vi "AIT 1553 - ReadWrite All Data.vi"(5 "Bus Section":T1, 6 "Iteration":i32, 7 "Mode":T2, 8 "error in (no error)":errorcluster, 11 "RT Data in":T3 {"Acyclic Frame Refs" format="%.0x"; "Label Transfer Config"."Block Data Refs"."Data Reference" format="%.0x"; "Status Config"."HWOut Dur Ref" format="%.0x"; "Status Config"."HWIn Dur Ref" format="%.0x"; "Status Config"."HWOut Count Ref" format="%.0x"; "Status Config"."HWIn Count Ref" format="%.0x"; "Status Config"."Error Data Ref" format="%.0x"; "HWOutput Channels"."Message Settings"."Driver Data"."First Word" min=8 max=31; "HWOutput Channels"."Message Settings"."Driver Data"."Num Bits" min=1 max=32; "HWOutput Channels"."Message Settings"."Driver Data"."Start Bit" min=8 max=31; "HWOutput Channels"."Message Settings"."Block Data Refs"."Data Reference" format="%.0x"; "HWInput Channels"."Message Settings"."Driver Data"."First Word" min=8 max=31; "HWInput Channels"."Message Settings"."Driver Data"."Num Bits" min=1 max=32; "HWInput Channels"."Message Settings"."Driver Data"."Start Bit" min=8 max=31; "HWInput Channels"."Message Settings"."Block Data Refs"."Data Reference" format="%.0x"}) -> (0 "error out":errorcluster, 3 "RT Data out":T3 {"Acyclic Frame Refs" format="%.0x"; "Label Transfer Config"."Block Data Refs"."Data Reference" format="%.0x"; "Status Config"."HWOut Dur Ref" format="%.0x"; "Status Config"."HWIn Dur Ref" format="%.0x"; "Status Config"."HWOut Count Ref" format="%.0x"; "Status Config"."HWIn Count Ref" format="%.0x"; "Status Config"."Error Data Ref" format="%.0x"; "HWOutput Channels"."Message Settings"."Driver Data"."First Word" min=8 max=31; "HWOutput Channels"."Message Settings"."Driver Data"."Num Bits" min=1 max=32; "HWOutput Channels"."Message Settings"."Driver Data"."Start Bit" min=8 max=31; "HWOutput Channels"."Message Settings"."Block Data Refs"."Data Reference" format="%.0x"; "HWInput Channels"."Message Settings"."Driver Data"."First Word" min=8 max=31; "HWInput Channels"."Message Settings"."Driver Data"."Num Bits" min=1 max=32; "HWInput Channels"."Message Settings"."Driver Data"."Start Bit" min=8 max=31; "HWInput Channels"."Message Settings"."Block Data Refs"."Data Reference" format="%.0x"})   [LabVIEW 2013, in "AIT 1553 Custom Device.lvlib"]
uses:
  AIT 1553 Custom Device.lvlib
  RT Controls/AIT 1553  - RT Data.ctl
  RT Controls/AIT 1553 - RT HW Channel.ctl
  RT Controls/AIT 1553 - Bus Section.ctl
  RT Controls/AIT 1553 - RT Message Settings.ctl
  <vilib>/NI Veristand/Custom Device API/Block Data Reference.ctl
  <vilib>/NI Veristand/Custom Device API/Data Reference.ctl
  RT Controls/AIT 1553 - Driver Data.ctl
  Controls and Global/Start Bit.ctl
  Controls and Global/Number of Bits.ctl
  RT Controls/AIT 1553 - Board Config Info.ctl
  RT Controls/AIT 1553 - Hardware Type.ctl
  RT Controls/Error Qs.ctl
  RT Controls/Status Channels Config.ctl
  RT Controls/FIFO.ctl
  RT Controls/Label Transfer Config.ctl
  <vilib>/NI Veristand/Custom Device API/Custom Device Item Ref.ctl
  RT Controls/ReadWrite Selector.ctl
  <vilib>/NI Veristand/Custom Device API/Custom Device API.lvlib
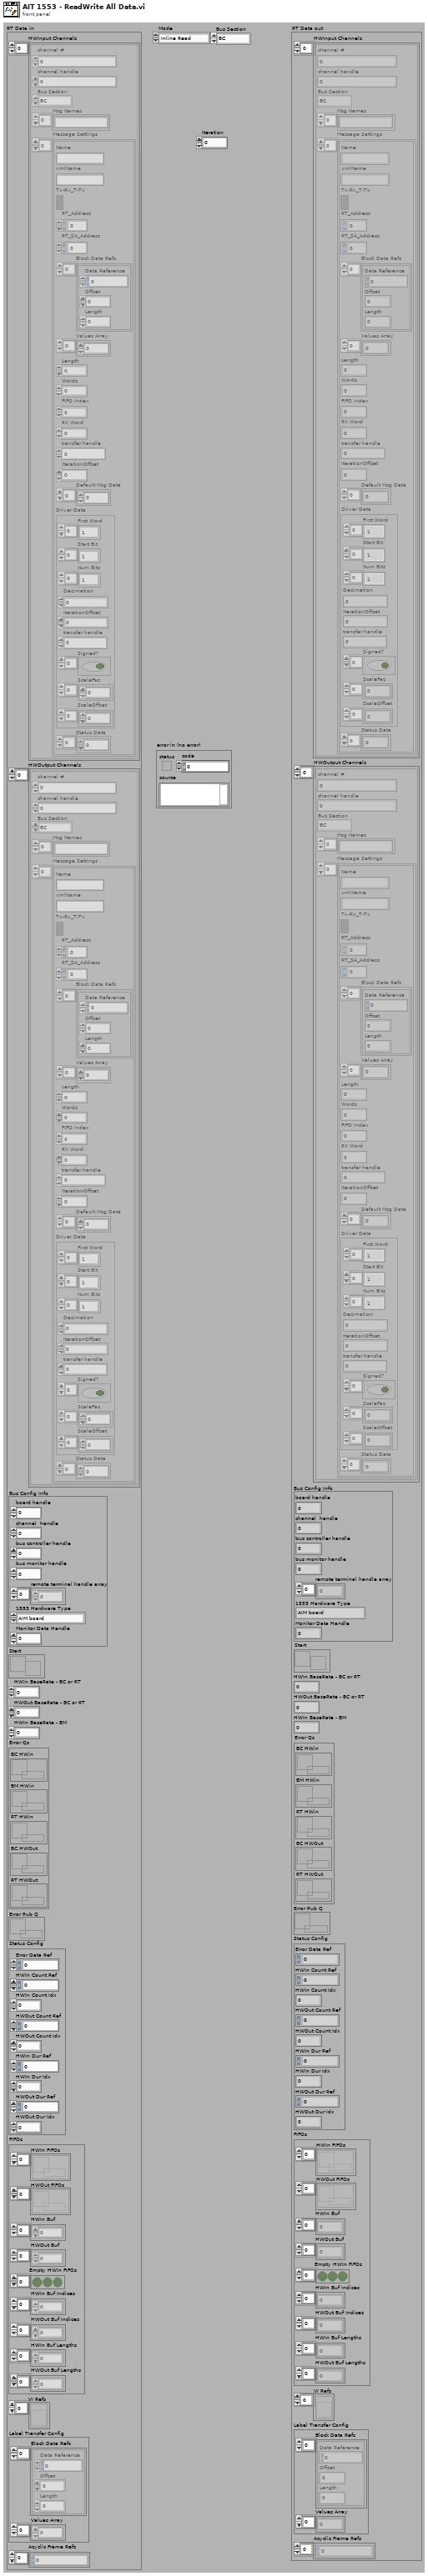
[diagram p1: front panel]
types:
  T1 = typedef "AIT 1553 Custom Device.lvlib/AIT 1553 - Bus Section.ctl" = enum16{"BC", "BM", "RT"}
  T2 = typedef "AIT 1553 Custom Device.lvlib/ReadWrite Selector.ctl" = enum16{"Inline Read", "Inline Write", "Async HWIn", "Async HWOut"}
  T3 = typedef "AIT 1553 Custom Device.lvlib/AIT 1553  - RT Data.ctl" = cluster{"HWInput Channels":T4[], "HWOutput Channels":T4[], "Bus Config Info":T11, "Start":refnum<notifier>, "HWIn BaseRate - BC or RT":i64, "HWOut BaseRate - BC or RT":i64, "HWIn BaseRate - BM":i64, "Error Qs":T13, "Error Pub Q":refnum<queue>, "Status Config":T14, "FIFOs":T15, "VI Refs":refnum<vi>[], "Label Transfer Config":T16, "Acyclic Frame Refs":T17[]}
  T4 = typedef "AIT 1553 Custom Device.lvlib/AIT 1553 - RT HW Channel.ctl" = cluster{"channel #":u16, "channel handle":u32, "Bus Section":T1, "Msg Names":string[], "Message Settings":T5[]}
  T5 = typedef "AIT 1553 Custom Device.lvlib/AIT 1553 - RT Message Settings.ctl" = cluster{"Name":string, "xmlName":string, "Tx-Rx_T-Tx":bool, "RT_Address":u8, "RT_SA_Address":u8, "Block Data Refs":T6[], "Values Array":dbl[], "Length":i32, "Words":i32, "FIFO Index":i32, "RX Word":u32, "transfer handle":u32, "IterationOffset":i32, "Default Msg Data":u16[], "Driver Data":T8, "Status Data":u32[]}
  T6 = typedef "Custom Device API.lvlib/Block Data Reference.ctl" = cluster{"Data Reference":T7, "Offset":i32, "Length":i32}
  T7 = typedef "Custom Device API.lvlib/Data Reference.ctl" = i32
  T8 = typedef "AIT 1553 Custom Device.lvlib/AIT 1553 - Driver Data.ctl" = cluster{"First Word":T9[], "Start Bit":T9[], "Num Bits":T10[], "Decimation":i32, "IterationOffset":i32, "transfer handle":u32, "Signed?":bool[], "ScaleFac":dbl[], "ScaleOffset":dbl[]}
  T9 = typedef "AIT 1553 Custom Device.lvlib/Start Bit.ctl" = i32
  T10 = typedef "AIT 1553 Custom Device.lvlib/Number of Bits.ctl" = i32
  T11 = typedef "AIT 1553 Custom Device.lvlib/AIT 1553 - Board Config Info.ctl" = cluster{"board handle":u32, "channel  handle":u32, "bus controller handle":u32, "bus monitor handle":u32, "remote terminal handle array":u32[], "1553 Hardware Type":T12, "Monitor Data Handle":u32}
  T12 = typedef "AIT 1553 Custom Device.lvlib/AIT 1553 - Hardware Type.ctl" = enum16{"AIM board", "AIT Board"}
  T13 = typedef "AIT 1553 Custom Device.lvlib/Error Qs.ctl" = cluster{"BC HWin":refnum<queue>, "BM HWin":refnum<queue>, "RT HWin":refnum<queue>, "BC HWOut":refnum<queue>, "RT HWOut":refnum<queue>}
  T14 = typedef "AIT 1553 Custom Device.lvlib/Status Channels Config.ctl" = cluster{"Error Data Ref":T7, "HWIn Count Ref":T7, "HWIn Count Idx":i32, "HWOut Count Ref":T7, "HWOut Count Idx":i32, "HWIn Dur Ref":T7, "HWIn Dur Idx":i32, "HWOut Dur Ref":T7, "HWOut Dur Idx":i32}
  T15 = typedef "AIT 1553 Custom Device.lvlib/FIFO.ctl" = cluster{"HWIn FIFOs":refnum<k33>[], "HWOut FIFOs":refnum<k33>[], "HWIn Buf":dbl[], "HWOut Buf":dbl[], "Empty HWIn FIFOs":bool[], "HWIn Buf Indices":i32[], "HWOut Buf Indices":i32[], "HWIn Buf Lengths":i32[], "HWOut Buf Lengths":i32[]}
  T16 = typedef "AIT 1553 Custom Device.lvlib/Label Transfer Config.ctl" = cluster{"Block Data Refs":T6[], "Values Array":dbl[]}
  T17 = typedef "Custom Device API.lvlib/Custom Device Item Ref.ctl" = u64
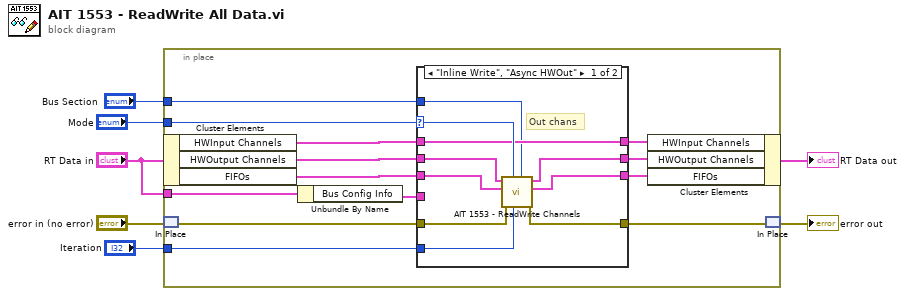
[diagram p0: block diagram]
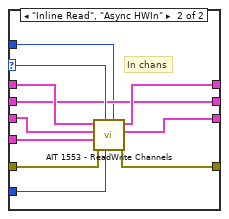
[diagram p2: hidden frame]
diagram:
  n1 = in-place {
    in-place-border: "Mode" -> [w14]
    in-place-border: "Bus Section" -> [w11]
    in-place-border: "Iteration" -> [w10]
    in-place-border: "RT Data in" -> [w9]
    n2 = in-place-cluster #1("RT Data in") -> ("HWInput Channels"=w20:T4[], "HWOutput Channels"=w13:T4[], "FIFOs"=w16:T15)
    n3 = in-place-match #2("error in (no error)") -> (w18:errorcluster)
    n4 = Unbundle By Name(w9) -> ("Bus Config Info"=w8:T11)
    n5 = case shown="\"Inline Write\", \"Async HWOut\"" w14 {
      selector: w14 -> [w29 w37]
      tunnel: w20 -> [w25 w41]
      tunnel: [w25 w40] -> w19
      tunnel: w18 -> [w30 w39]
      tunnel: [w28 w38] -> w17
      tunnel: w16 -> [w23 w35]
      tunnel: [w24 w34] -> w15
      tunnel: w13 -> [w27 w36]
      tunnel: [w26 w36] -> w12
      tunnel: w11 -> [w22 w33]
      tunnel: w10 -> [w21 w32]
      tunnel: w8 -> [_ w31]
      frame "Inline Write", "Async HWOut" {
        # "Out chans"
        n6 = call "AIT 1553 - ReadWrite Channels.vi"("Bus Section"=w22, "Iteration"=w21, "Mode"=w29, "error in (no error)"=w30, "FIFOs In"=w23, "Channels In"=w27) -> ("error out"=w28:errorcluster, "FIFOs Out"=w24:T15, "Channels Out"=w26:T4[])  [unwired: 3 in]
      }
      frame "Inline Read", "Async HWIn" {
        # "In chans"
        n7 = call "AIT 1553 - ReadWrite Channels.vi"("Bus Section"=w33, "Iteration"=w32, "Mode"=w37, "error in (no error)"=w39, "Bus Config Info"=w31, "FIFOs In"=w35, "Channels In"=w41) -> ("error out"=w38:errorcluster, "FIFOs Out"=w34:T15, "Channels Out"=w40:T4[])  [unwired: 2 in]
      }
    }
    n8 = in-place-cluster #1("HWInput Channels"=w19, "HWOutput Channels"=w12, "FIFOs"=w15) -> (→"RT Data out":T3)
    n9 = in-place-match #2(w17) -> (→"error out":errorcluster)
  }
